vi "upackConfigVars.vi"(11 "file":path) -> (2 "configJSON":T1)   [LabVIEW 2017]
panel:
  out "result string":string
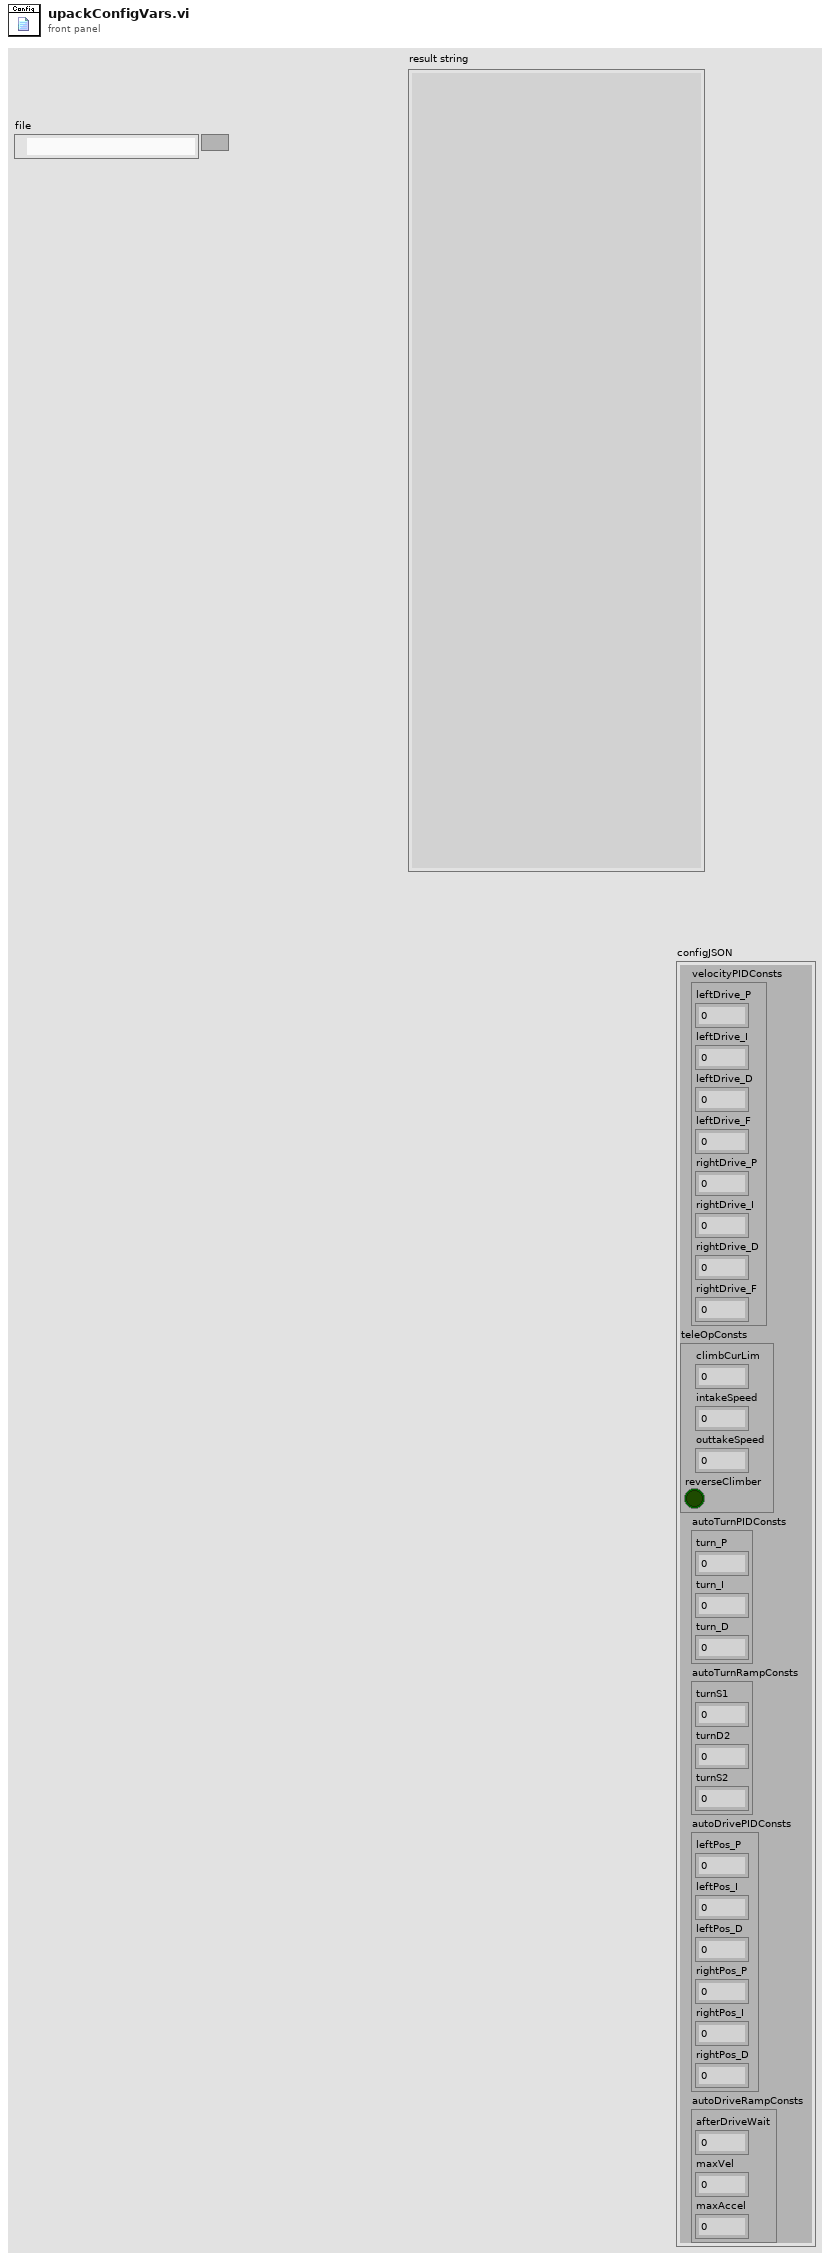
[diagram p1: front panel]
types:
  T1 = cluster{"velocityPIDConsts":cluster{"leftDrive_P":dbl, "leftDrive_I":dbl, "leftDrive_D":dbl, "leftDrive_F":dbl, "rightDrive_P":dbl, "rightDrive_I":dbl, "rightDrive_D":dbl, "rightDrive_F":dbl}, "teleOpConsts":cluster{"climbCurLim":dbl, "intakeSpeed":dbl, "outtakeSpeed":dbl, "reverseClimber":bool}, "autoTurnPIDConsts":cluster{"turn_P":dbl, "turn_I":dbl, "turn_D":dbl}, "autoTurnRampConsts":cluster{"turnS1":dbl, "turnD2":dbl, "turnS2":dbl}, "autoDrivePIDConsts":cluster{"leftPos_P":dbl, "leftPos_I":dbl, "leftPos_D":dbl, "rightPos_P":dbl, "rightPos_I":dbl, "rightPos_D":dbl}, "autoDriveRampConsts":cluster{"afterDriveWait":dbl, "maxVel":dbl, "maxAccel":dbl}}
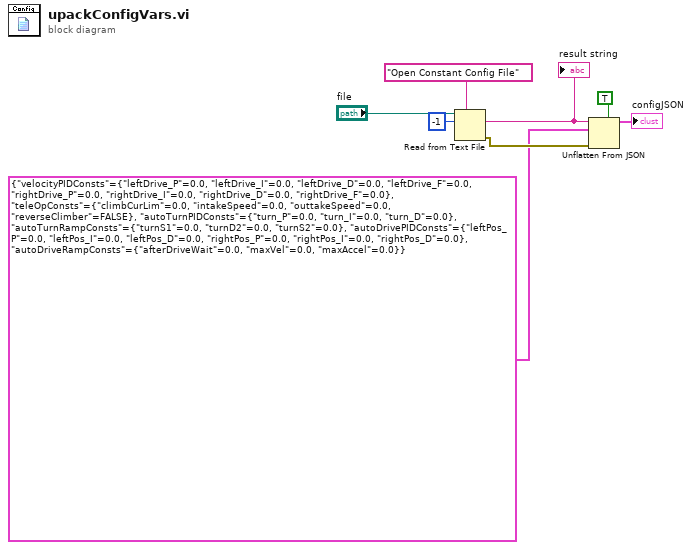
[diagram p0: block diagram]
diagram:
  n1 = Read from Text File(prompt (Open existing file)="Open Constant Config File", file (use dialog)="file", count=-1) -> (text=w4:string, error out=w3:errorcluster)  [unwired: 1 in, 2 out]
  "result string" <- w4
  n2 = Unflatten From JSON(enable LabVIEW extensions? (T)=TRUE, JSON string=w4, type and defaults=T1 {"velocityPIDConsts"={"leftDrive_P"=0.0, "leftDrive_I"=0.0, "leftDrive_D"=0.0, "leftDrive_F"=0.0, "rightDrive_P"=0.0, "rightDrive_I"=0.0, "rightDrive_D"=0.0, "rightDrive_F"=0.0}, "teleOpConsts"={"climbCurLim"=0.0, "intakeSpeed"=0.0, "outtakeSpeed"=0.0, "reverseClimber"=FALSE}, "autoTurnPIDConsts"={"turn_P"=0.0, "turn_I"=0.0, "turn_D"=0.0}, "autoTurnRampConsts"={"turnS1"=0.0, "turnD2"=0.0, "turnS2"=0.0}, "autoDrivePIDConsts"={"leftPos_P"=0.0, "leftPos_I"=0.0, "leftPos_D"=0.0, "rightPos_P"=0.0, "rightPos_I"=0.0, "rightPos_D"=0.0}, "autoDriveRampConsts"={"afterDriveWait"=0.0, "maxVel"=0.0, "maxAccel"=0.0}}, error in (no error)=w3) -> (value=→"configJSON":T1)  [unwired: 3 in, 1 out]
